vi "Dequeue Next Song.vi"(8 "error in (no error)":errorcluster, 11 "SongQueueActor In":refnum<class "SongQueueActor.lvclass">) -> (0 "error out":errorcluster, 3 "SongQueueActor Out":refnum<class "SongQueueActor.lvclass">)   [LabVIEW 2015, in "SongQueueActor.lvlib" / "SongQueueActor.lvclass"]
uses:
  SongQueueActor.lvclass
  SongQueueActor.lvclass/SongQueueActor.ctl
  file/MusicElement/MusicElementLibrary/MusicElementLibrary.lvclass/MusicElementLibrary.ctl
  controls/Queue Song Display.ctl
  file/MusicElement/Song/Song Duration.ctl
  controls/Dequeue Control.ctl
  builds/xctls/Song Queue/Song Queue.lvlibp/app/xctls/SongQueue/Song Queue.xctl
  file/MusicElement/MusicElement.lvclass
  SongPlayerActor/SongPlayerActor Messages/Play Song Msg/Play Song Msg.lvclass
  file/MusicElement/Song/Song.lvclass
  file/MusicElement/MusicElementLibrary/MusicElementLibrary.lvclass
  AlbumImageActor/AlbumImageActor Messages/Download Album Image Msg/Download Album Image Msg.lvclass
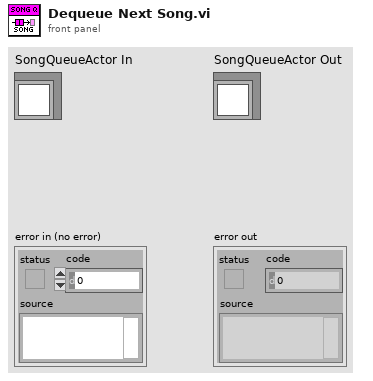
[diagram p1: front panel]
types:
  T1 = typedef "Queue Song Display.ctl" = cluster{"Song Name":string, "Artist":string, "Album":string, "Duration (s)":T2, "UID":string, "Dequeue":T3}
  T2 = typedef "Song.lvclass/Song Duration.ctl" = timestamp
  T3 = typedef "Dequeue Control.ctl" = bool
  T4 = typedef "Song Queue.lvlibp/Queue Song Display.ctl" = cluster{"Song Name":string, "Artist":string, "Album":string, "Duration (s)":T5, "UID":string, "Dequeue":T6}
  T5 = typedef "Song Queue.lvlibp/Song.lvclass/Song Duration.ctl" = timestamp
  T6 = typedef "Song Queue.lvlibp/Dequeue Control.ctl" = bool
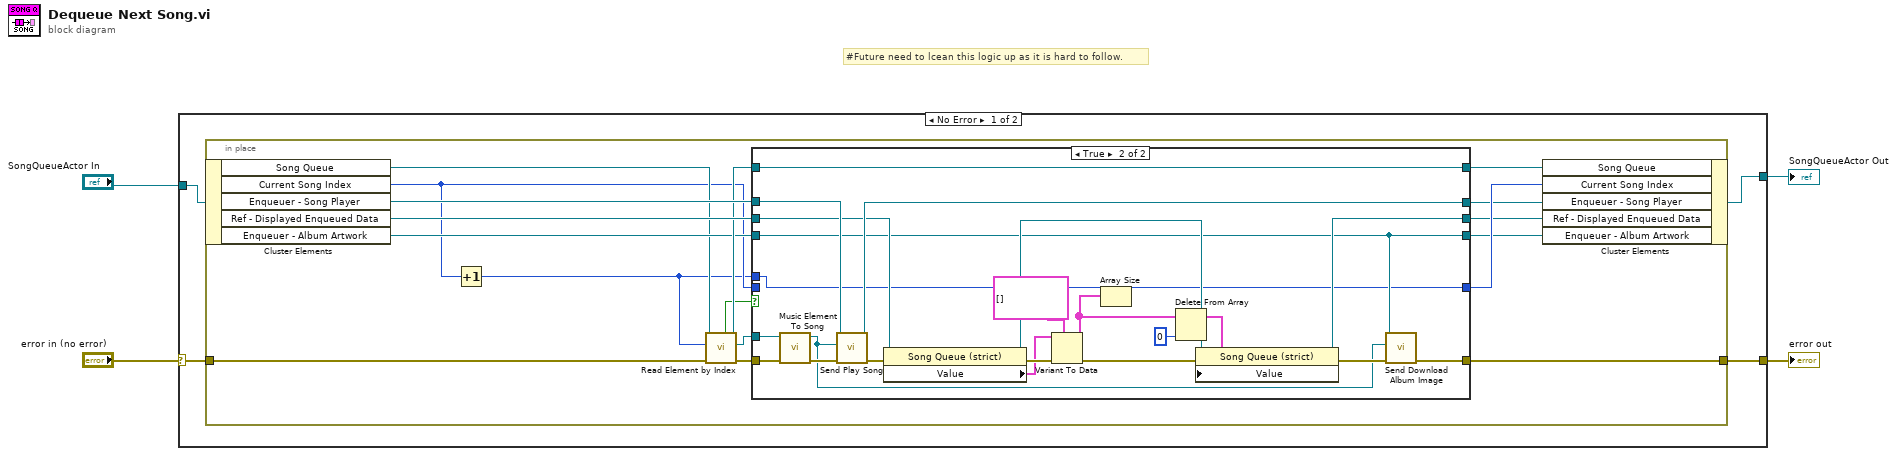
[diagram p0: block diagram]
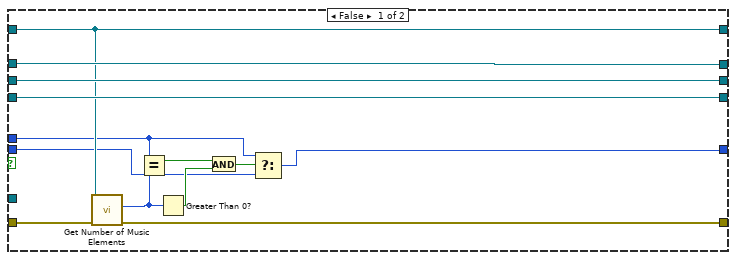
[diagram p2: hidden frame]
diagram:
  # "#Future need to lcean this logic up as it is hard to follow."
  n1 = case shown="No Error" "error in (no error)" {
    selector: "error in (no error)" -> [w7 w62]
    tunnel: [w5 w62] -> w3
    tunnel: [w6 w61] -> w2
    tunnel: "SongQueueActor In" -> [w8 w61]
    frame No Error {
      n2 = in-place {
        in-place-border: w7 -> [w10]
        in-place-border: [w22] -> w5
        n3 = in-place-cluster #1(w8) -> ("Song Queue"=w12:refnum<class "SongLibrary.lvclass">, "Current Song Index"=w11:i32, "Enqueuer - Song Player"=w24:refnum<class "Message Enqueuer.lvclass">, "Ref - Displayed Enqueued Data"=w21:refnum<vi>, "Enqueuer - Album Artwork"=w14:refnum<class "Message Enqueuer.lvclass">)
        n4 = Increment(x=w11) -> (x+1=w9:i32)
        n5 = call "Read Element by Index.vi"("error in (no error)"=w10, "index"=w9, "MusicElementLibrary in"=w12) -> ("error out"=w16:errorcluster, "MusicElement.lvclass"=w15:refnum<class "MusicElement.lvclass">, "MusicElementLibrary out"=w18:refnum<class "SongLibrary.lvclass">, "Found?"=w17:bool)  [unwired: 5 in]
        n6 = case shown="True" w17 {
          tunnel: w11 -> [w26 _]
          tunnel: [w32 w39] -> w25
          tunnel: w16 -> [w34 w46]
          tunnel: w24 -> [w38 w60]
          tunnel: [w38 w59] -> w23
          tunnel: [w33 w42] -> w22
          tunnel: w21 -> [w37 w52]
          tunnel: [w37 w49] -> w20
          tunnel: [w35 w47] -> w19
          tunnel: w18 -> [w35 w47]
          tunnel: w15 -> [_ w44]
          tunnel: w14 -> [w36 w40]
          tunnel: [w36 w40] -> w13
          tunnel: w9 -> [w27 w39]
          frame False {
            n7 = call "Get Number of Music Elements.vi"("error in (no error)"=w34, "MusicElementLibrary in"=w35) -> ("error out"=w33:errorcluster, "Size"=w31:i32)  [unwired: 7 in, 1 out]
            n8 = Equal?(x=w27, y=w31) -> (x = y?=w29:bool)
            n9 = Greater Than 0?(x=w31) -> (x > 0?=w28:bool)
            n10 = And(x=w29, y=w28) -> (x .and. y?=w30:bool)
            n11 = Select(t=w27, s=w30, f=w26) -> (s? t:f=w32:i32)
          }
          frame True {
            n12 = call "Music Element To Song.vi"("error in (no error)"=w46, "MusicElement"=w44) -> ("error out"=w45:errorcluster, "Song out"=w41:refnum<class "Song.lvclass">)  [unwired: 8 in]
            n13 = call "Send Play Song.vi"("error in (no error)"=w45, "Song"=w41, "Message Enqueuer in"=w60) -> ("error out"=w53:errorcluster, "Message Enqueuer out"=w59:refnum<class "Message Enqueuer.lvclass">)  [unwired: 7 in]
            n14 = property class="Song Queue (strict)"(reference=w52, error in=w53) -> (reference out=w51:refnum<vi>, error out=w58:errorcluster, "Value"=w57:T4[])
            n15 = Variant To Data(error in=w58, type=T1[] [], Variant=w57) -> (data=w55:T1[], error out=w50:errorcluster)
            n16 = Array Size(array=w55) -> ()  [unwired: 1 out]
            n17 = Delete From Array(array=w55, index=0) -> (array with subset deleted=w54:T1[])  [unwired: 1 in, 1 out]
            n18 = property class="Song Queue (strict)"(reference=w51, error in=w50, "Value"=w54) -> (reference out=w49:refnum<vi>, error out=w43:errorcluster)
            n19 = call "Send Download Album Image.vi"("error in (no error)"=w43, "Song"=w41, "Message Enqueuer in"=w40) -> ("error out"=w42:errorcluster)  [unwired: 7 in, 1 out]
          }
        }
        n20 = in-place-cluster #1("Song Queue"=w19, "Current Song Index"=w25, "Enqueuer - Song Player"=w23, "Ref - Displayed Enqueued Data"=w20, "Enqueuer - Album Artwork"=w13) -> (w6:refnum<class "SongQueueActor.lvclass">)
      }
    }
    frame Error {
    }
  }
  "error out" <- w3
  "SongQueueActor Out" <- w2
